vi "Untitled 4.vi"() -> (1 "j":i32, 2 "i":i32)   [LabVIEW 2024]
panel:
  out "j 2":i32
  out "i 2":i32
  in  "stop":bool
  in  "Array":bool[][](array[boolean])
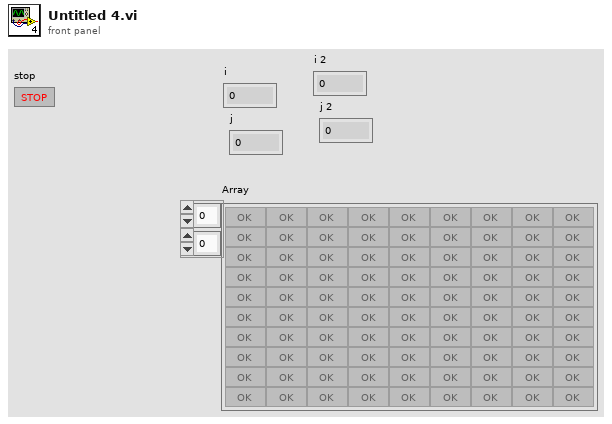
[diagram p1: front panel]
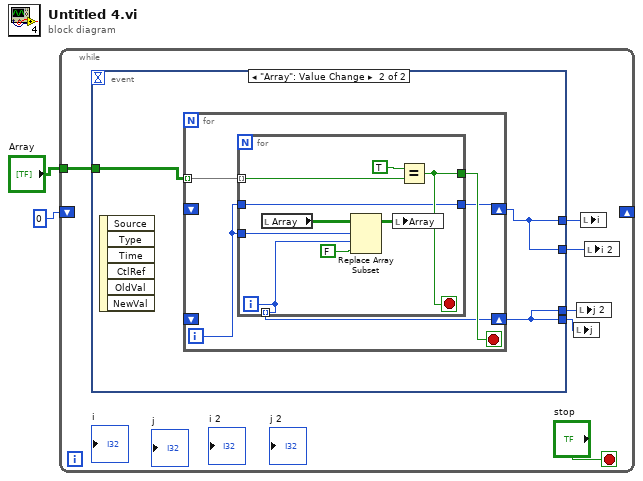
[diagram p0: block diagram]
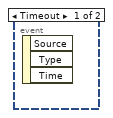
[diagram p2: hidden frame]
diagram:
  n1 = while {
    shift-right: _ -> [_]
    shift-left: 0 -> [_]
    tunnel: "Array" -> [w3]
    stop <- "stop" stop-if-true
    n2 = event shown="[1] \"Array\": Value Change" {
      selector: _ -> [_ _]
      dyn-events: _ -> [_ _]
      timeout: _ -> [_ _]
      tunnel: [_ w11] -> w7
      tunnel: [_ w11] -> w6
      tunnel: [_ w10] -> w5
      tunnel: [_ w10] -> w4
      tunnel: w3 -> [_ w9]
      event Timeout {
        n3 = event-data() -> ()  [unwired: 1 in, 3 out]
      }
      event "Array": Value Change {
        n4 = event-data() -> ()  [unwired: 1 in, 6 out]
        n5 = for {
          tunnel: w9 -> [w16] mode=indexing
          shift-right: [w13] -> w11
          shift-left: _ -> [_]
          shift-right: [w12] -> w10
          shift-left: _ -> [_]
          i -> [w14]
          stop <- w15 stop-if-true
          n6 = for {
            tunnel: w16 -> [w25] mode=indexing
            tunnel: [w23] -> w15
            tunnel: w14 -> [w18]
            tunnel: w14 -> [w20]
            tunnel: [w17] -> w12
            tunnel: [w18] -> w13
            tunnel: [w17] -> _ mode=indexing
            i -> [w17]
            stop <- w23 stop-if-true
            n7 = local read "Array"() -> (w22:bool[][])
            n8 = Replace Array Subset(array=w22, new element=FALSE ("new element/subarray"), index (row)=w20, index (col)=w17) -> (w21:bool[][])
            n9 = local write "Array"(w21) -> ()
            n10 = Equal?(x=TRUE, y=w25) -> (x = y?=w23:bool)
          }
        }
      }
    }
    n11 = local write "j"(w5) -> ()
    n12 = local write "j 2"(w4) -> ()
    n13 = local write "i"(w7) -> ()
    n14 = local write "i 2"(w6) -> ()
  }
